vi "FindMax.vi"(0 "Algorithm":enum16{"RRT", "A*"}(ring), 4 "k":i32=1, 6 "Depth":i32=1, 8 "KD Tree":dbl[][](array[numeric]), 9 "Dim":i32=1, 10 "index":i32) -> (2 "Max Node":dbl[](array[numeric]))   [LabVIEW 2016]
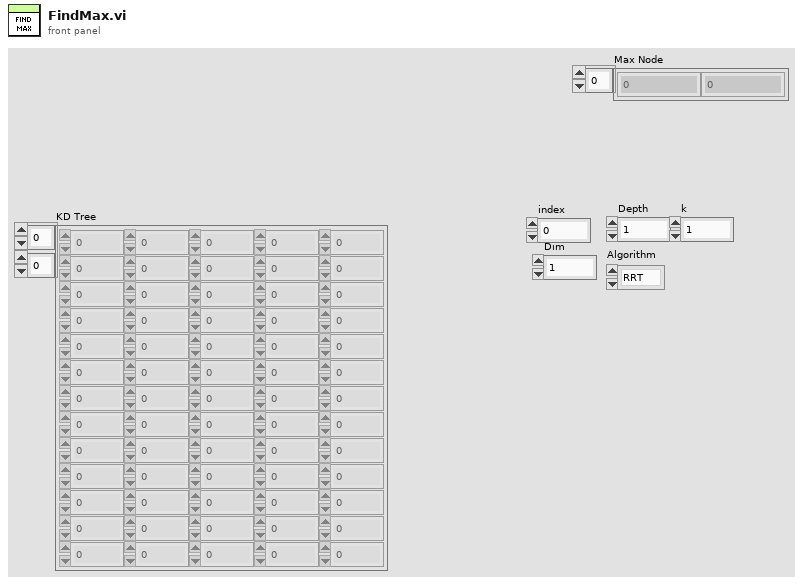
[diagram p1: front panel]
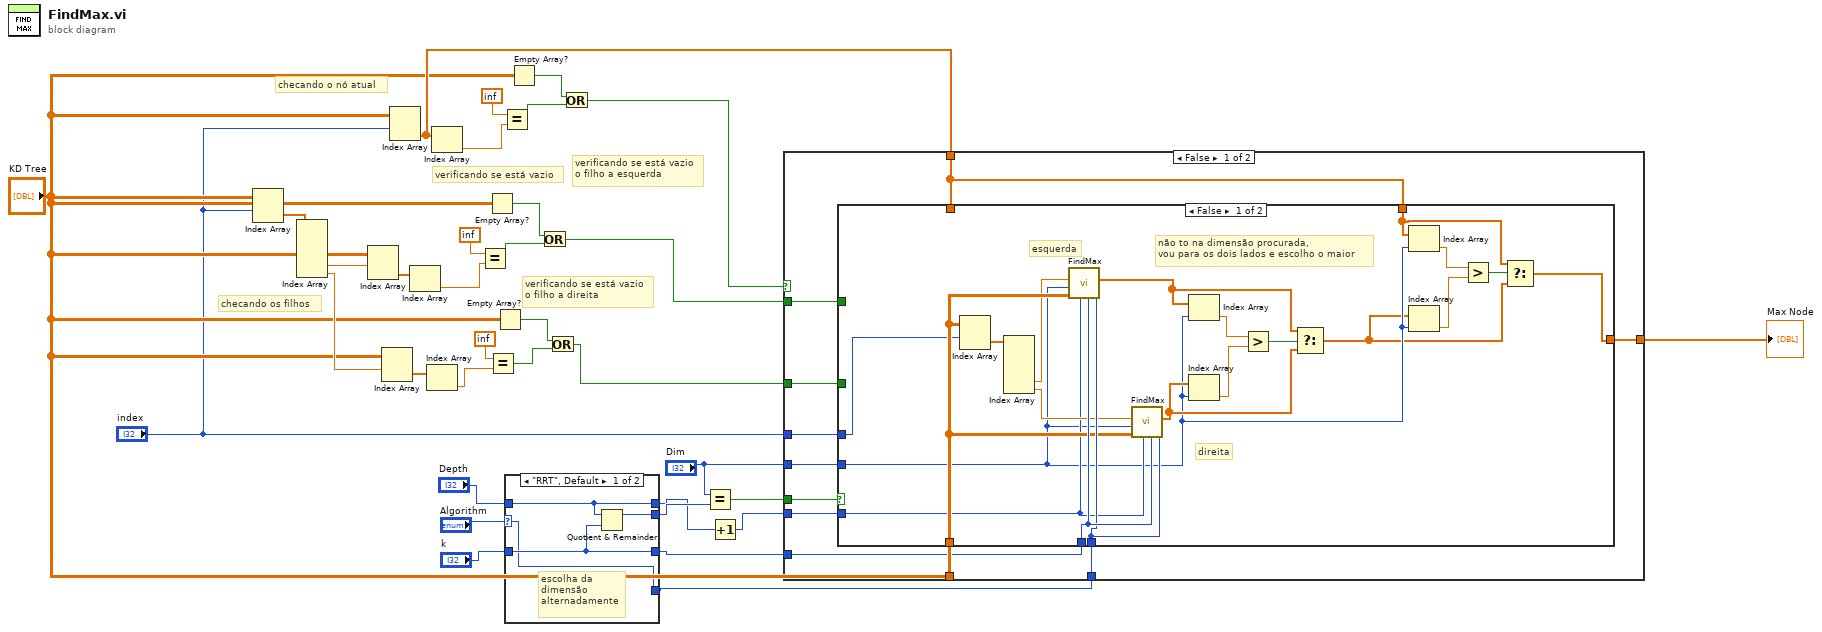
[diagram p0: block diagram]
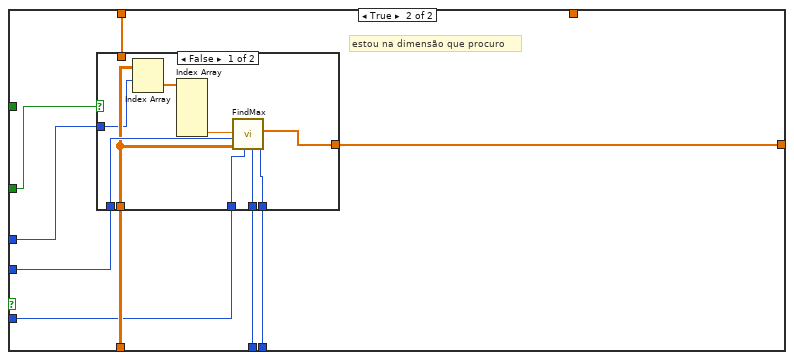
[diagram p2: hidden frame]
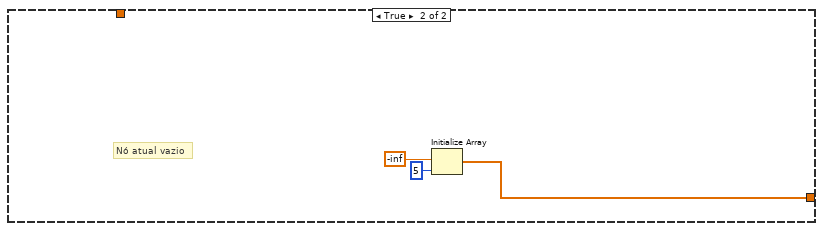
[diagram p4: hidden frame]
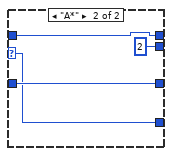
[diagram p5: hidden frame]
diagram:
  # "verificando se está vazio\no filho a direita"
  # "checando o nó atual"
  # "verificando se está vazio"
  # "verificando se está vazio\no filho a esquerda"
  # "checando os filhos"
  n1 = Index Array(array="KD Tree", index (row)="index") -> (element=w19:dbl[])  [unwired: 1 in]
  n2 = Index Array(array=w19) -> (element #4=w28:dbl, element #5=w24:dbl)  [unwired: 5 in, 3 out]
  n3 = Index Array(array="KD Tree", index (row)=w28) -> (element=w23:dbl[])  [unwired: 1 in]
  n4 = Index Array(array="KD Tree", index (row)=w24) -> (element=w21:dbl[])  [unwired: 1 in]
  n5 = Index Array(array="KD Tree", index (row)="index") -> (element=w9:dbl[])  [unwired: 1 in]
  n6 = Index Array(array=w23) -> (element=w22:dbl)  [unwired: 1 in]
  n7 = Index Array(array=w21) -> (element=w20:dbl)  [unwired: 1 in]
  n8 = Index Array(array=w9) -> (element=w13:dbl)  [unwired: 1 in]
  n9 = Equal?(x=inf, y=w22) -> (x = y?=w29:bool)
  n10 = Empty Array?(array="KD Tree") -> (empty?=w30:bool)
  n11 = Equal?(x=inf, y=w20) -> (x = y?=w25:bool)
  n12 = Empty Array?(array="KD Tree") -> (empty?=w26:bool)
  n13 = Equal?(x=inf, y=w13) -> (x = y?=w14:bool)
  n14 = case shown="\"RRT\", Default" "Algorithm" {
    selector: "Algorithm" -> [w35 w39]
    tunnel: [w38 2] -> w18
    tunnel: [w37 w40] -> w2
    tunnel: [w36 w42] -> w4
    tunnel: "Depth" -> [w37 w40]
    tunnel: "k" -> [w36 w42]
    tunnel: [w35 w39] -> w3
    frame "RRT", Default {
      # "escolha da \ndimensão \nalternadamente"
      n15 = Quotient & Remainder(x=w37, y=w36) -> (x-y*floor(x/y)=w38:i32)  [unwired: 1 out]
    }
    frame "A*" {
    }
  }
  n16 = Empty Array?(array="KD Tree") -> (empty?=w15:bool)
  n17 = Or(x=w30, y=w29) -> (x .or. y?=w11:bool)
  n18 = Or(x=w26, y=w25) -> (x .or. y?=w10:bool)
  n19 = Or(x=w15, y=w14) -> (x .or. y?=w12:bool)
  n20 = Equal?(x="Dim", y=w18) -> (x = y?=w17:bool)
  n21 = Increment(x=w2) -> (x+1=w1:i32)
  n22 = case shown="False" w12 {
    tunnel: w17 -> [w53 _]
    tunnel: w11 -> [w52 _]
    tunnel: w10 -> [w51 _]
    tunnel: w9 -> [w43 _]
    tunnel: [w50 w93] -> w8
    tunnel: "KD Tree" -> [w49 _]
    tunnel: "Dim" -> [w48 _]
    tunnel: "index" -> [w47 _]
    tunnel: w4 -> [w46 _]
    tunnel: w3 -> [w45 _]
    tunnel: w1 -> [w44 _]
    frame False {
      n23 = case shown="False" w53 {
        tunnel: w52 -> [_ _]
        tunnel: w51 -> [_ w74]
        tunnel: w43 -> [_ w82]
        tunnel: [w54 w81] -> w50
        tunnel: w49 -> [w66 w80]
        tunnel: w48 -> [w58 w79]
        tunnel: w47 -> [w65 w78]
        tunnel: w46 -> [w68 w77]
        tunnel: w45 -> [w67 w76]
        tunnel: w44 -> [w61 w75]
        tunnel: w43 -> [w55 _]
        frame False {
          # "direita"
          # "esquerda"
          # "não to na dimensão procurada, \nvou para os dois lados e escolho o maior"
          n24 = Index Array(array=w66, index (row)=w65) -> (element=w64:dbl[])  [unwired: 1 in]
          n25 = Index Array(array=w64) -> (element #4=w63:dbl, element #5=w62:dbl)  [unwired: 5 in, 3 out]
          n26 = call "FindMax.vi"("Algorithm"=w67, "k"=w68, "Depth"=w61, "KD Tree"=w66, "Dim"=w58, "index"=w63) -> ("Max Node"=w70:dbl[])  [unwired: 5 in]
          n27 = call "FindMax.vi"("Algorithm"=w67, "k"=w68, "Depth"=w61, "KD Tree"=w66, "Dim"=w58, "index"=w62) -> ("Max Node"=w69:dbl[])  [unwired: 5 in]
          n28 = Index Array(array=w70, index=w58) -> (element=w73:dbl)
          n29 = Index Array(array=w69, index=w58) -> (element=w72:dbl)
          n30 = Greater?(x=w73, y=w72) -> (0:w71:bool)
          n31 = Select(t=w70, s=w71, f=w69) -> (s? t:f=w56:dbl[])
          n32 = Index Array(array=w55, index=w58) -> (element=w60:dbl)
          n33 = Index Array(array=w56, index=w58) -> (element=w57:dbl)
          n34 = Greater?(x=w60, y=w57) -> (0:w59:bool)
          n35 = Select(t=w55, s=w59, f=w56) -> (s? t:f=w54:dbl[])
        }
        frame True {
          # "estou na dimensão que procuro"
          n36 = case shown="False" w74 {
            tunnel: w82 -> [_ w92]
            tunnel: [w91 w92] -> w81
            tunnel: w80 -> [w88 _]
            tunnel: w79 -> [w89 _]
            tunnel: w78 -> [w87 _]
            tunnel: w77 -> [w84 _]
            tunnel: w76 -> [w86 _]
            tunnel: w75 -> [w85 _]
            frame False {
              n37 = Index Array(array=w88, index (row)=w87) -> (element=w90:dbl[])  [unwired: 1 in]
              n38 = Index Array(array=w90) -> (element #5=w83:dbl)  [unwired: 5 in, 4 out]
              n39 = call "FindMax.vi"("Algorithm"=w86, "k"=w84, "Depth"=w85, "KD Tree"=w88, "Dim"=w89, "index"=w83) -> ("Max Node"=w91:dbl[])  [unwired: 5 in]
            }
            frame True {
              # "n tem nada a direita"
            }
          }
        }
      }
    }
    frame True {
      # "Nó atual vazio"
      n40 = Initialize Array(-inf, 5 ("dimension size")) -> (w93:dbl[])
    }
  }
  "Max Node" <- w8
